vi "test-cubic-spline-01.vi"() -> ()   [LabVIEW 2019]
uses:
  <vilib>/Rock Robotics/WPI/ThirdParty/JAS_Junk/TrajLib/POSEwCURVATURE.ctl
  <vilib>/Rock Robotics/WPI/ThirdParty/JAS_Junk/TrajLib/POSE2D.ctl
  <vilib>/Rock Robotics/WPI/ThirdParty/JAS_Junk/TrajLib/TRANSLATION2D.ctl
  <vilib>/Rock Robotics/WPI/ThirdParty/JAS_Junk/TrajLib/ROTATION2D.ctl
  <vilib>/Rock Robotics/WPI/ThirdParty/JAS_Junk/TrajLib/Rotation_CreateAngle.vi
  <vilib>/Rock Robotics/WPI/ThirdParty/JAS_Junk/TrajLib/Util_CalcDist.vi
  <vilib>/Rock Robotics/WPI/ThirdParty/JAS_Junk/TrajLib/Trajectory_Library.lvlib
panel:
  out "All Interior \nwayPoints\nFound (True)":bool
  out "end rot = 0":dbl
  out "end y = 0":dbl
  out "end x = 0":dbl
  out "start rot = 0":dbl
  out "start y = 0":dbl
  out "start x = 0":dbl
  out "max dtheta < 0.0872":dbl
  out "max dy < 0.00127":dbl
  out "max dx  < 0.127":dbl
  out "Overall Error":errorcluster
  out "Elements":i32
  out "Create Spline Error":errorcluster
  out "SplinePoses\nWCurve":T1[](array[typedef]) {"POSE"."ROTATION"."SIN" format="%13.4f"; "POSE"."ROTATION"."COS" format="%13.4f"; "POSE"."ROTATION"."VALUE" format="%13.4f"; "POSE"."TRANSLATION"."Y" format="%14.3f"; "POSE"."TRANSLATION"."X" format="%14.3f"}
  out "Elapsed Time":dbl
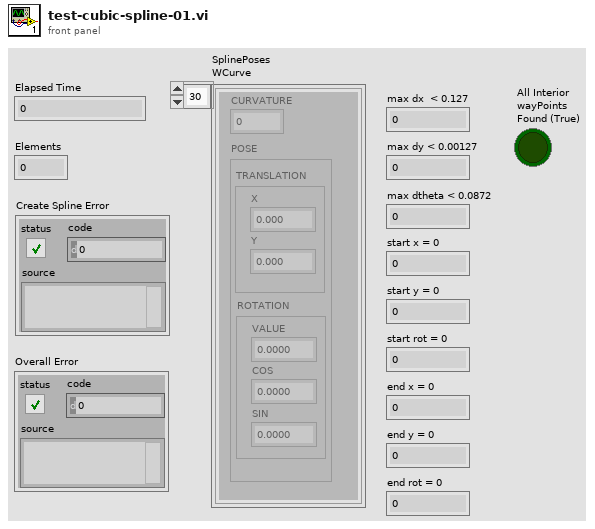
[diagram p1: front panel]
types:
  T1 = typedef "Trajectory_Library.lvlib/POSEwCURVATURE.ctl" = cluster{"CURVATURE":dbl, "POSE":T2}
  T2 = typedef "Trajectory_Library.lvlib/POSE2D.ctl" = cluster{"TRANSLATION":T3, "ROTATION":T4}
  T3 = typedef "Trajectory_Library.lvlib/TRANSLATION2D.ctl" = cluster{"X":dbl, "Y":dbl}
  T4 = typedef "Trajectory_Library.lvlib/ROTATION2D.ctl" = cluster{"VALUE":dbl, "COS":dbl, "SIN":dbl}
  T5 = typedef "Trajectory_Library.lvlib/SPLINE_CTRL_VECTOR.ctl" = cluster{"Xs":dbl[], "Ys":dbl[]}
  T6 = typedef "Trajectory_Library.lvlib/SPLINE.ctl" = cluster{"Degree":i32, "Coefficients":T7}
  T7 = typedef "NI_Matrix.lvlib/RealMatrix.ctl" = dbl[][]
  T8 = typedef "Trajectory_Library.lvlib/TWIST2D.ctl" = cluster{"dX":dbl, "dY":dbl, "dTHETA":dbl}
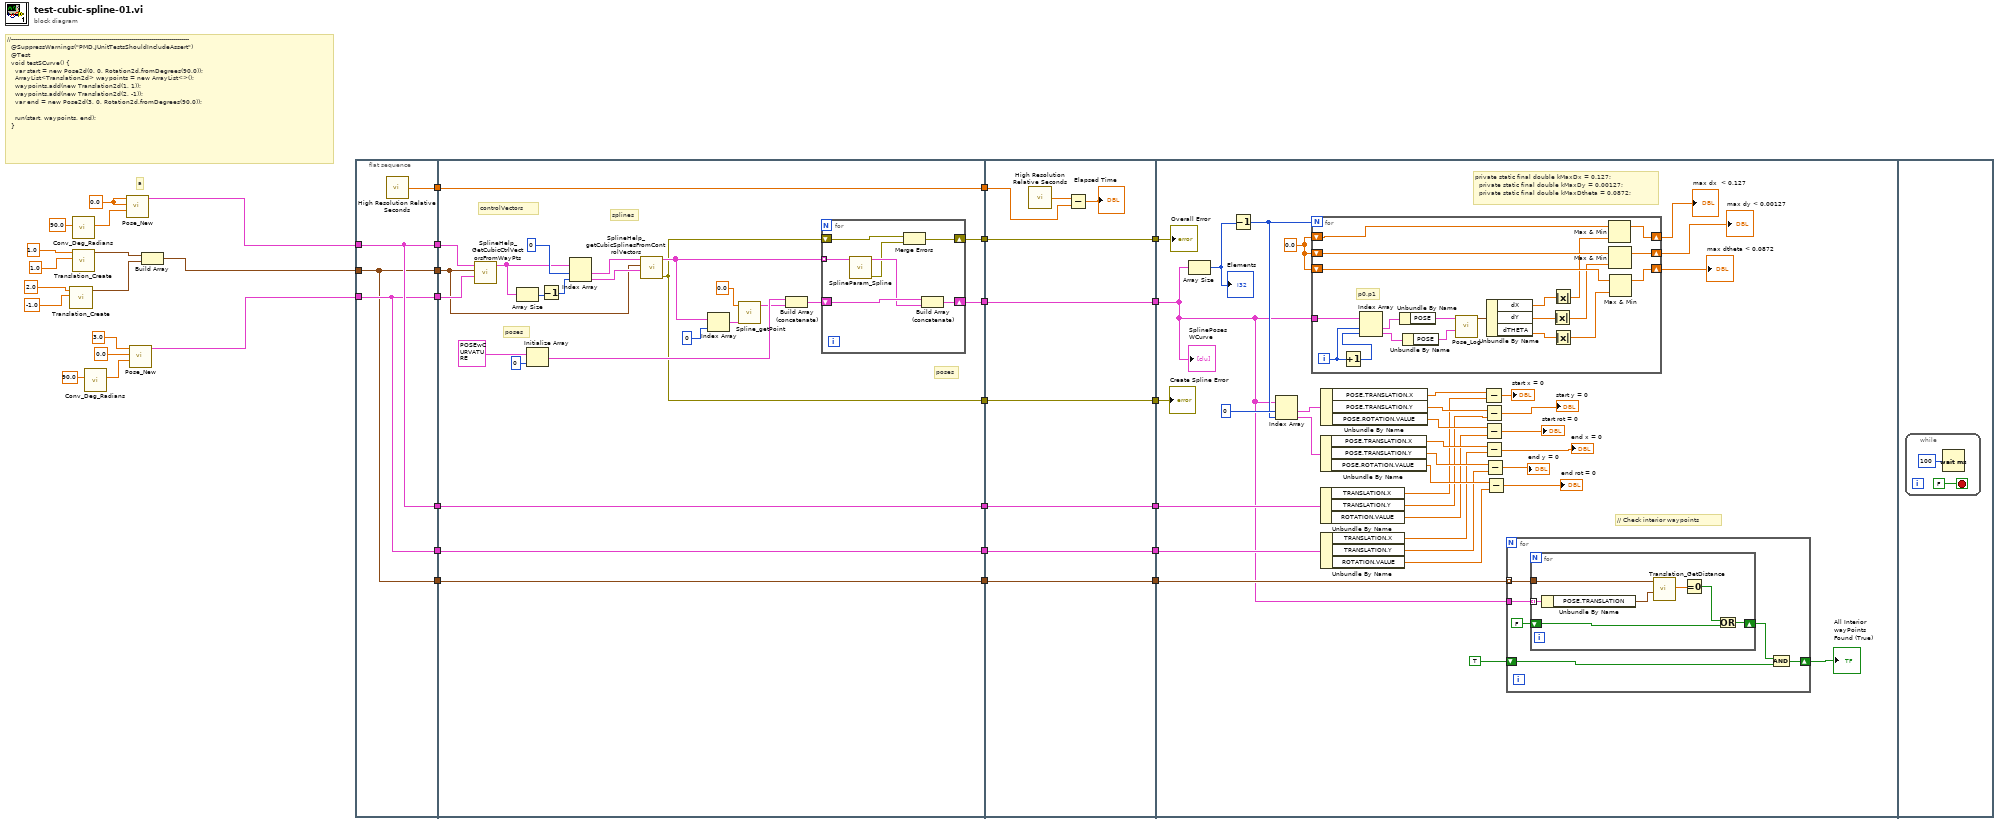
[diagram p0: block diagram]
diagram:
  w12 = 0.0 ("X")
  # "a"
  # "//-----------------------------------------------------------------------------------------\n  @SuppressWarnings(\"PMD.JUnitTestsShouldIncludeAssert\")\n  @Test\n  void testSCurve() {\n    var start = new Pose2d(0, 0, Rotation2d.fromDegrees(90.0));\n    ArrayList<Translation2d> waypoints = new ArrayList<>();\n    waypoints.add(new Translation2d(1, 1));\n    waypoints.add(new Translation2d(2, -1));\n    var end = new Pose2d(3, 0, Rotation2d.fromDegrees(90.0));\n\n    run(start, waypoints, end);\n  }"
  n1 = call <vilib>:"Translation_Create.vi"("Y"=-1.0, "X"=2.0) -> ("TRANSLATION"=w7:T3)  [unwired: 9 in]
  n2 = call <vilib>:"Conv_Deg_Radians.vi"("Degress"=90.0) -> ("Radians"=w11:dbl)  [unwired: 10 in]
  n3 = call <vilib>:"Translation_Create.vi"("Y"=1.0, "X"=1.0) -> ("TRANSLATION"=w8:T3)  [unwired: 9 in]
  n4 = call <vilib>:"Conv_Deg_Radians.vi"("Degress"=90.0) -> ("Radians"=w1:dbl)  [unwired: 10 in]
  n5 = call <vilib>:"Pose_New.vi"("Heading"=w11, "Y"=w12, "X"=w12) -> ("out POSe"=w34:T2)  [unwired: 8 in]
  n6 = call <vilib>:"Pose_New.vi"("Heading"=w1, "Y"=0.0, "X"=3.0) -> ("out POSe"=w31:T2)  [unwired: 8 in]
  n7 = Build Array(w8, w7) -> (w9:T3[])
  n8 = flat-sequence {
    tunnel: w34 -> [w39]
    tunnel: [w39] -> w33
    tunnel: w9 -> [w37]
    tunnel: [w37] -> w32
    tunnel: w31 -> [w38]
    tunnel: [w38] -> w30
    tunnel: [w40] -> w29
    tunnel: [w39] -> w21
    tunnel: [w38] -> w18
    tunnel: [w37] -> w13
    tunnel: w33 -> [w65]
    tunnel: w32 -> [w57]
    tunnel: w30 -> [w64]
    tunnel: [w56] -> w28
    tunnel: w29 -> [w56]
    tunnel: [w46] -> w27
    tunnel: [w45] -> w25
    tunnel: [w44] -> w23
    tunnel: w21 -> [w43]
    tunnel: [w43] -> w20
    tunnel: w18 -> [w42]
    tunnel: [w42] -> w17
    tunnel: [w41] -> w14
    tunnel: w13 -> [w41]
    tunnel: w28 -> [w81]
    tunnel: w27 -> [w80]
    tunnel: [w80] -> w26
    tunnel: w25 -> [w79]
    tunnel: [w79] -> w24
    tunnel: w23 -> [w78]
    tunnel: [w78] -> w22
    tunnel: w20 -> [w75]
    tunnel: [w75] -> w19
    tunnel: w17 -> [w74]
    tunnel: [w74] -> w16
    tunnel: [w73] -> w15
    tunnel: w14 -> [w73]
    tunnel: w26 -> [w84]
    tunnel: w24 -> [w116]
    tunnel: w22 -> [w115]
    tunnel: w19 -> [w109]
    tunnel: w16 -> [w108]
    tunnel: w15 -> [w85]
    frame #0 {
      n9 = call <vilib>:"High Resolution Relative Seconds.vi"() -> ("relative seconds"=w40:dbl)
    }
    frame #1 {
      # "poses"
      # "poses"
      # "splines"
      # "controlVectors"
      n10 = call <vilib>:"SplineHelp_GetCubicCtrlVectorsFromWayPts.vi"("Enging POSE"=w64, "Interior WAYPOINTS"=w57, "Starting POSE"=w65) -> ("SplineControlVectors"=w61:T5[])  [unwired: 8 in]
      n11 = Array Size(array=w61) -> (size(s)=w62:i32)
      n12 = Initialize Array(T1 {"CURVATURE"=0.0, "POSE"={"TRANSLATION"={"X"=0.0, "Y"=0.0}, "ROTATION"={"VALUE"=0.0, "COS"=1.0, "SIN"=0.0}}} ("POSEwCURVATURE"), 0 ("dimension size")) -> (w50:T1[])
      n13 = Decrement(x=w62) -> (x-1=w60:i32)
      n14 = Index Array(array=w61, index #1=0 ("index"), index #2=w60) -> (element #1=w59:T5, element #2=w58:T5)
      n15 = call <vilib>:"SplineHelp_getCubicSplinesFromControlVectors.vi"("endCtrlVector"=w58, "InternalWaypoints"=w57, "startCtrlVector"=w59) -> ("error out"=w45:errorcluster, "splines"=w47:T6[])  [unwired: 3 in, 4 out]
      n16 = Index Array(array=w47, index=0) -> (element=w52:T6)
      n17 = call <vilib>:"Spline_getPoint.vi"("inputSPLINE"=w52, "Time"=0.0) -> ("POSEwCURVATURE"=w49:T1)  [unwired: 9 in]
      n18 = Build Array (concatenate)(w50, w49) -> (w48:T1[])
      n19 = for {
        shift-right: [w69] -> w46
        shift-left: w48 -> [w71]
        tunnel: w47 -> [w72] mode=indexing
        shift-right: [w67] -> w44
        shift-left: w45 -> [w68]
        n20 = call <vilib>:"SplineParam_Spline.vi"("inputSPLINE"=w72) -> ("error out"=w66:errorcluster, "outputPOSEwCURVATURE"=w70:T1[])  [unwired: 9 in]
        n21 = Merge Errors(w68, w66) -> (w67:errorcluster)
        n22 = Build Array (concatenate)(w71, w70) -> (w69:T1[])
      }
    }
    frame #2 {
      n23 = call <vilib>:"High Resolution Relative Seconds.vi"() -> ("relative seconds"=w76:dbl)
      n24 = Subtract(x=w76, y=w81) -> (x-y=→"Elapsed Time":dbl)
    }
    frame #3 {
      w113 = 0.0
      # "// Check interior waypoints"
      # "private static final double kMaxDx = 0.127;\n  private static final double kMaxDy = 0.00127;\n  private static final double kMaxDtheta = 0.0872;"
      n25 = Array Size(array=w84) -> (size(s)=w114:i32)
      "Elements" <- w114
      n26 = Decrement(x=w114) -> (x-1=w106:i32)
      n27 = Index Array(array=w84, index #1=0 ("index"), index #2=w106) -> (element #1=w105:T1, element #2=w104:T1)
      n28 = for {
        N: w106 -> [_]
        tunnel: w84 -> [w147]
        shift-right: [w138] -> w112
        shift-left: w113 -> [w135]
        shift-right: [w136] -> w110
        shift-left: w113 -> [w133]
        shift-right: [w137] -> w111
        shift-left: w113 -> [w134]
        i -> [w149]
        # "p0,p1"
        n29 = Increment(x=w149) -> (x+1=w148:i32)
        n30 = Index Array(array=w147, index #1=w149, index #2=w148) -> (element #1=w146:T1, element #2=w145:T1)
        n31 = Unbundle By Name(w146) -> ("POSE"=w144:T2)
        n32 = Unbundle By Name(w145) -> ("POSE"=w143:T2)
        n33 = call <vilib>:"Pose_Log.vi"("end POSE"=w143, "in POSE"=w144) -> ("out TWIST"=w142:T8)  [unwired: 9 in]
        n34 = Unbundle By Name(w142) -> ("dX"=w139:dbl, "dY"=w140:dbl, "dTHETA"=w141:dbl)
        n35 = Absolute Value(x=w140) -> (abs(x)=w131:dbl)
        n36 = Absolute Value(x=w139) -> (abs(x)=w132:dbl)
        n37 = Absolute Value(x=w141) -> (abs(x)=w130:dbl)
        n38 = Max & Min(x=w135, y=w132) -> (max(x,y)=w138:dbl)  [unwired: 1 out]
        n39 = Max & Min(x=w134, y=w131) -> (max(x,y)=w137:dbl)  [unwired: 1 out]
        n40 = Max & Min(x=w133, y=w130) -> (max(x,y)=w136:dbl)  [unwired: 1 out]
      }
      "max dx  < 0.127" <- w112
      "max dy < 0.00127" <- w111
      "max dtheta < 0.0872" <- w110
      n41 = Unbundle By Name(w104) -> ("POSE.TRANSLATION.X"=w100:dbl, "POSE.TRANSLATION.Y"=w99:dbl, "POSE.ROTATION.VALUE"=w98:dbl)
      n42 = Unbundle By Name(w109) -> ("TRANSLATION.X"=w97:dbl, "TRANSLATION.Y"=w96:dbl, "ROTATION.VALUE"=w95:dbl)
      n43 = Unbundle By Name(w105) -> ("POSE.TRANSLATION.X"=w103:dbl, "POSE.TRANSLATION.Y"=w102:dbl, "POSE.ROTATION.VALUE"=w101:dbl)
      n44 = Unbundle By Name(w108) -> ("TRANSLATION.X"=w94:dbl, "TRANSLATION.Y"=w93:dbl, "ROTATION.VALUE"=w92:dbl)
      n45 = Subtract(x=w103, y=w97) -> (x-y=→"start x = 0":dbl)
      n46 = Subtract(x=w102, y=w96) -> (x-y=→"start y = 0":dbl)
      n47 = Subtract(x=w101, y=w95) -> (x-y=→"start rot = 0":dbl)
      n48 = Subtract(x=w100, y=w94) -> (x-y=→"end x = 0":dbl)
      n49 = Subtract(x=w99, y=w93) -> (x-y=→"end y = 0":dbl)
      n50 = Subtract(x=w98, y=w92) -> (x-y=→"end rot = 0":dbl)
      n51 = for {
        tunnel: w85 -> [w117] mode=indexing
        tunnel: w84 -> [w122]
        shift-right: [w121] -> w82
        shift-left: TRUE -> [w120]
        n52 = for {
          tunnel: w122 -> [w126] mode=indexing
          shift-right: [w129] -> w118
          shift-left: FALSE -> [w128]
          tunnel: w117 -> [w127]
          n53 = Unbundle By Name(w126) -> ("POSE.TRANSLATION"=w125:T3)
          n54 = call <vilib>:"Translation_GetDistance.vi"("other Translation"=w125, "In Translation"=w127) -> ("Distance"=w124:dbl)  [unwired: 9 in]
          n55 = Equal To 0?(x=w124) -> (x = 0?=w123:bool)
          n56 = Or(x=w123, y=w128) -> (x .or. y?=w129:bool)
        }
        n57 = And(x=w118, y=w120) -> (x .and. y?=w121:bool)
      }
      "All Interior \nwayPoints\nFound (True)" <- w82
      "SplinePoses\nWCurve" <- w84
      "Create Spline Error" <- w116
      "Overall Error" <- w115
    }
    frame #4 {
      n58 = while {
        stop <- FALSE stop-if-true
        n59 = Wait (ms)(milliseconds to wait=u32 100) -> ()  [unwired: 1 out]
      }
    }
  }
